vi "Configure Common PUSCH Allocation.vi"(0 "VISA resource name":refnum<visa-resource-name>, 1 "Mapping Type (A)":i32(ring) items=["A", "B"], 2 "Start Symbol (0)":i32, 3 "No RBs (1)":i32=1, 5 "Instance (1)":T3=1, 7 "CC (1)":T2=1, 9 "Allocation (1)":T1=1, 10 "Modulation Scheme (Pi/2-BPSK)":i32(ring) items=["Pi/2-BPSK", "QPSK", "16-QAM", "64-QAM", "256-QAM", "Pi/2-BPSK with shaping"], 11 "error in (no error)":errorcluster, 12 "No Symbols (4)":i32=4, 13 "Auto Detect (Off)":bool, 14 "Start RB (0)":i32) -> (4 "VISA resource name out":refnum<visa-resource-name>, 15 "error out":errorcluster)   [LabVIEW 2020, in "Rohde&Schwarz CMWXP NR FR1 Measurement.lvlib"]
doc: "Specifies settings related to the PUSCH allocation, for carrier <no>, allocation <a>.\n\nAttribute:\nRSCMWXPNRFR1M_ATTR_COMMON_PUSCH_ALLOCATION\n\nRemote-control command:\nCONFigure:NRSub:MEAS<i>[:CC<no>]:ALLocation<a>:PUSCh"
uses:
  <instrlib>/Rohde&Schwarz CMWXP NR FR1 Measurement/Rohde&Schwarz CMWXP NR FR1 Measurement.lvlib
  <instrlib>/Rohde&Schwarz CMWXP NR FR1 Measurement/Private/_Instance.ctl
  <instrlib>/Rohde&Schwarz CMWXP NR FR1 Measurement/Private/_Carrier Component.ctl
  <instrlib>/Rohde&Schwarz CMWXP NR FR1 Measurement/Private/_Allocation.ctl
  <instrlib>/Rohde&Schwarz CMWXP NR FR1 Measurement/Private/rsidr_core.llb/rsidr_core.lvlib
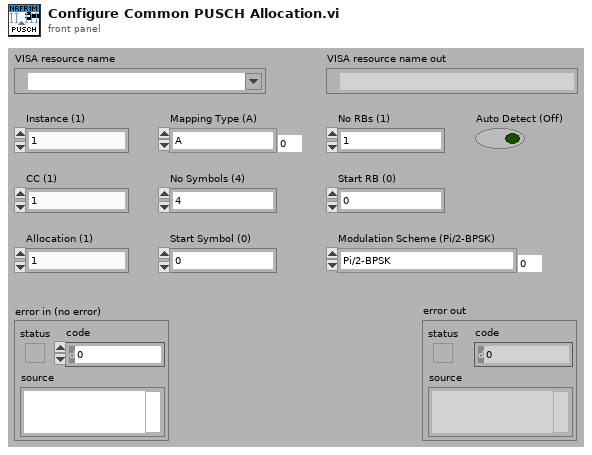
[diagram p1: front panel]
types:
  T1 = typedef "Rohde&Schwarz CMWXP NR FR1 Measurement.lvlib/_Allocation.ctl" = i32
  T2 = typedef "Rohde&Schwarz CMWXP NR FR1 Measurement.lvlib/_Carrier Component.ctl" = i32
  T3 = typedef "Rohde&Schwarz CMWXP NR FR1 Measurement.lvlib/_Instance.ctl" = i32
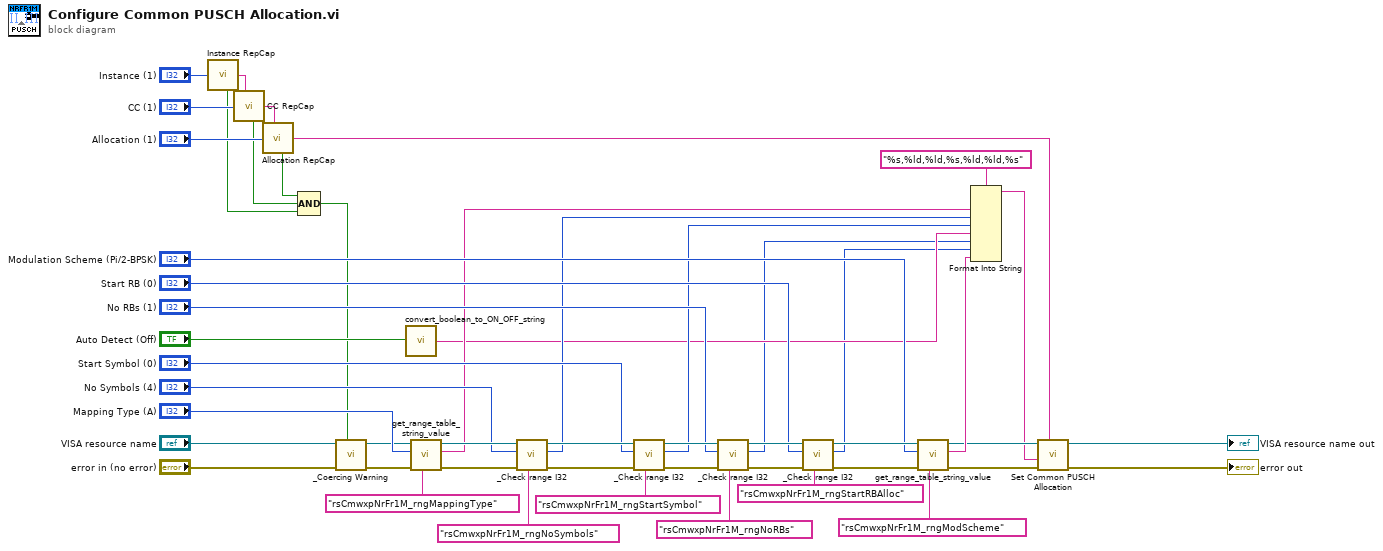
[diagram p0: block diagram]
diagram:
  n1 = call <instrlib>:"Instance RepCap.vi"("Instance In"="Instance (1)") -> ("In Range?"=w2:bool, "RepCap Identifier Out"=w45:string)  [unwired: 1 in]
  n2 = call <instrlib>:"CC RepCap.vi"("CC In"="CC (1)", "RepCap String In (\"\")"=w45) -> ("In Range?"=w3:bool, "RepCap Identifier Out"=w44:string)
  n3 = call <instrlib>:"Allocation RepCap.vi"("Allocation In"="Allocation (1)", "RepCap String In (\"\")"=w44) -> ("In Range?"=w4:bool, "RepCap Identifier Out"=w43:string)
  n4 = Compound Arithmetic op=AND(w4, w3, w2) -> (w1:bool)
  n5 = call <instrlib>:"_Coercing Warning.vi"("In Range?"=w1, "error in (no error)"="error in (no error)", "VISA resource name"="VISA resource name") -> ("error out"=w6:errorcluster, "VISA resource name out"=w5:refnum<visa-resource-name>)  [unwired: 7 in]
  n6 = call <instrlib>:"convert_boolean_to_ON_OFF_string.vi"("boolean value in"="Auto Detect (Off)") -> ("string value out"=w15:string)  [unwired: 4 in]
  n7 = call <instrlib>:"get_range_table_string_value.vi"("Range Table ID in"="rsCmwxpNrFr1M_rngMappingType", "error in"=w6, "I32 input"="Mapping Type (A)", "VISA resource name"=w5) -> ("error out"=w40:errorcluster, "String Value out"=w18:string, "VISA resource name out"=w39:refnum<visa-resource-name>)  [unwired: 5 in]
  n8 = call <instrlib>:"_Check range I32.vi"("Range Table Identifier"="rsCmwxpNrFr1M_rngNoSymbols", "error in (no error)"=w40, "I32 Value In"="No Symbols (4)", "VISA resource name"=w39) -> ("error out"=w36:errorcluster, "I32 Value Out"=w17:i32, "VISA resource name out"=w35:refnum<visa-resource-name>)  [unwired: 5 in]
  n9 = call <instrlib>:"_Check range I32.vi"("Range Table Identifier"="rsCmwxpNrFr1M_rngStartSymbol", "error in (no error)"=w36, "I32 Value In"="Start Symbol (0)", "VISA resource name"=w35) -> ("error out"=w31:errorcluster, "I32 Value Out"=w16:i32, "VISA resource name out"=w30:refnum<visa-resource-name>)  [unwired: 5 in]
  n10 = call <instrlib>:"_Check range I32.vi"("Range Table Identifier"="rsCmwxpNrFr1M_rngNoRBs", "error in (no error)"=w31, "I32 Value In"="No RBs (1)", "VISA resource name"=w30) -> ("error out"=w27:errorcluster, "I32 Value Out"=w14:i32, "VISA resource name out"=w26:refnum<visa-resource-name>)  [unwired: 5 in]
  n11 = call <instrlib>:"_Check range I32.vi"("Range Table Identifier"="rsCmwxpNrFr1M_rngStartRBAlloc", "error in (no error)"=w27, "I32 Value In"="Start RB (0)", "VISA resource name"=w26) -> ("error out"=w22:errorcluster, "I32 Value Out"=w13:i32, "VISA resource name out"=w21:refnum<visa-resource-name>)  [unwired: 5 in]
  n12 = call <instrlib>:"get_range_table_string_value.vi"("Range Table ID in"="rsCmwxpNrFr1M_rngModScheme", "error in"=w22, "I32 input"="Modulation Scheme (Pi/2-BPSK)", "VISA resource name"=w21) -> ("error out"=w11:errorcluster, "String Value out"=w12:string, "VISA resource name out"=w10:refnum<visa-resource-name>)  [unwired: 5 in]
  n13 = Format Into String(format string="%s,%ld,%ld,%s,%ld,%ld,%s", w18, w17, w16, w15, w14, w13, w12) -> (resulting string=w9:string)  [unwired: 2 in, 1 out]
  n14 = call "Set Common PUSCH Allocation"("Repeated Capabilities"=w43, "error in (no error)"=w11, "Common PUSCH Allocation ()"=w9, "instrument handle"=w10) -> ("error out"=→"error out":errorcluster, "instrument handle out"=→"VISA resource name out":refnum<visa-resource-name>)  [unwired: 6 in]
